vi "SimAcq.vi"(8 "error in (no error)":errorcluster, 11 "Instruments in":refnum<class "Instruments.lvclass">) -> (0 "error out":errorcluster, 3 "Instruments out":refnum<class "Instruments.lvclass">)   [LabVIEW 2012, in "Instruments.lvclass"]
uses:
  Instruments.lvclass
  Controls/TestData.ctl
  Controls/Measurement.ctl
  Controls/CurrentPad.ctl
  Controls/PadArea.ctl
  <userlib>/_OpenG.lib/numeric/numeric.llb/Random Number Within Range - DBL__ogtk.vi
panel:
  in  "Value":T1
  out "TestData":T3 {"50mA Data"."Reverse" format="%#_3g"; "50mA Data"."Current,mA" format="%_6g"; "50mA Data"."Knee Current" format="%#_3g"; "50mA Data"."WL" format="%_6g"; "50mA Data"."Voltage" format="%_6g"; "50mA Data"."Power" format="%_5g"; "20mA Data"."Reverse" format="%#_3g"; "20mA Data"."Current,mA" format="%_6g"; "20mA Data"."Knee Current" format="%#_3g"; "20mA Data"."WL" format="%_6g"; "20mA Data"."Voltage" format="%_6g"; "20mA Data"."Power" format="%_5g"}
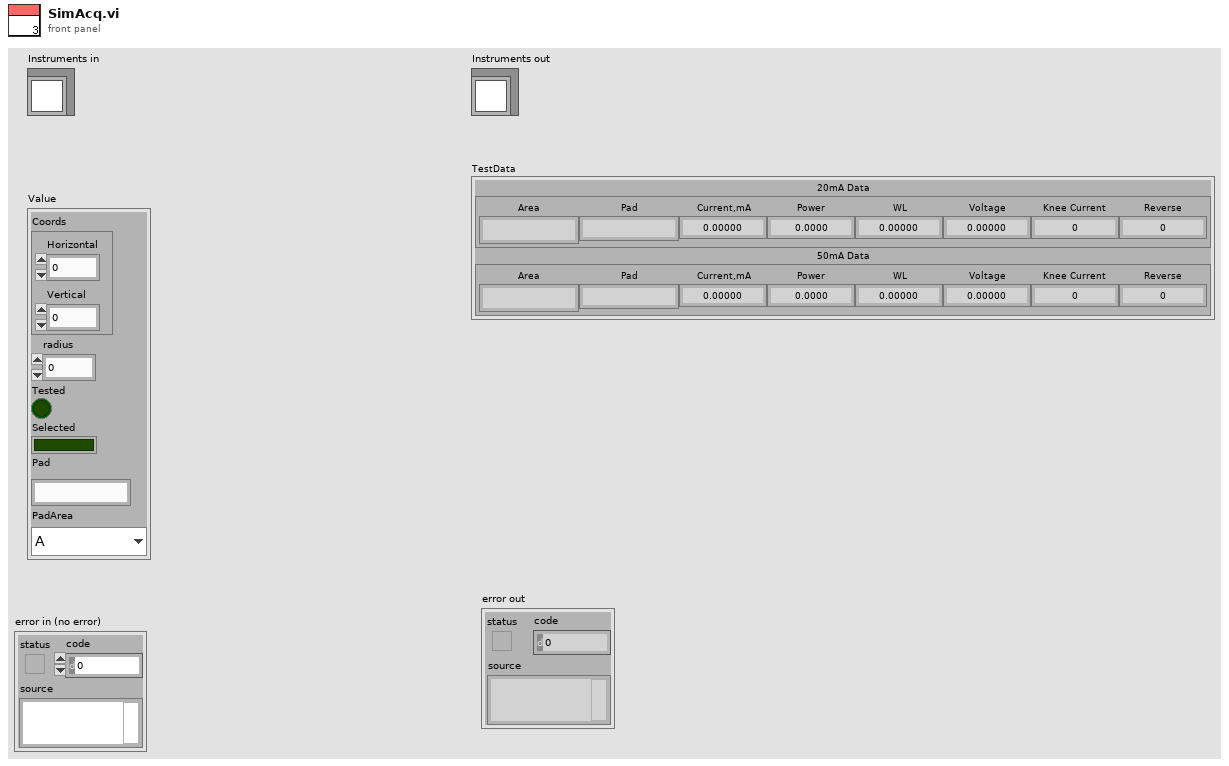
[diagram p1: front panel]
types:
  T1 = typedef "CurrentPad.ctl" = cluster{"Coords":cluster{"Horizontal":sgl, "Vertical":sgl}, "radius":i32, "Tested":bool, "Selected":bool, "Pad":string, "PadArea":T2}
  T2 = typedef "PadArea.ctl" = enum16{"A", "B", "C", "D", "L", "R", "T", "G"}
  T3 = typedef "TestData.ctl" = cluster{"20mA Data":T4, "50mA Data ":T4}
  T4 = typedef "Measurement.ctl" = cluster{"Area":string, "Pad":string, "Current,mA":dbl, "Power":dbl, "WL":dbl, "Voltage":dbl, "Knee Current":dbl, "Reverse":dbl}
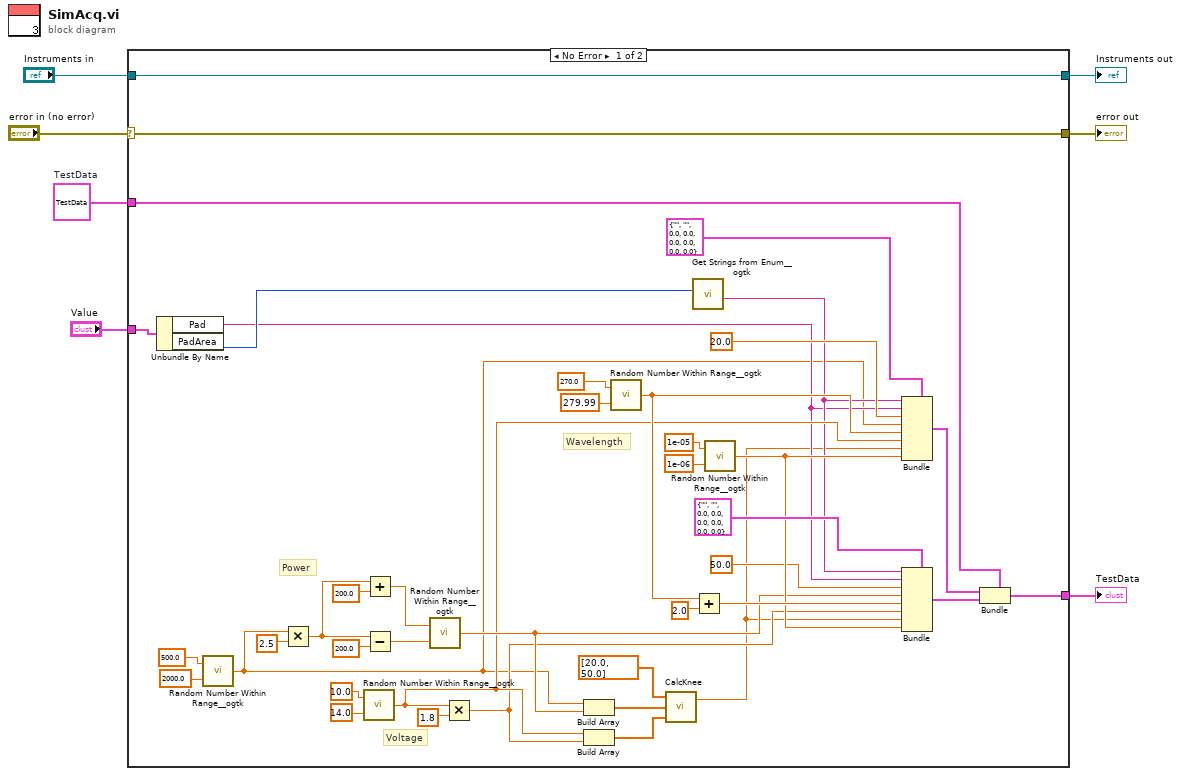
[diagram p0: block diagram]
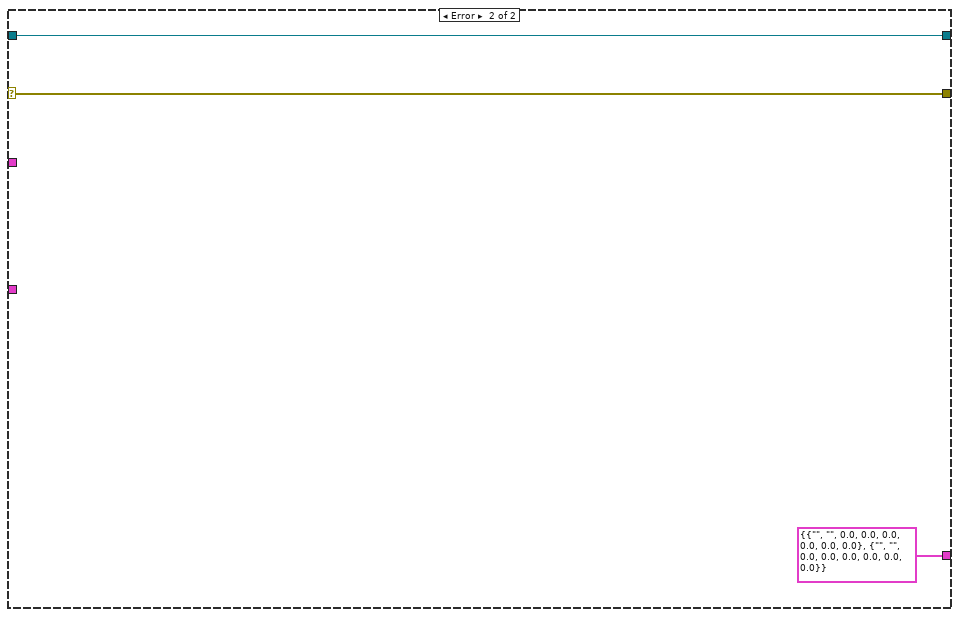
[diagram p2: hidden frame]
diagram:
  w3 = T3 {"20mA Data"={"Area"="", "Pad"="", "Current,mA"=0.0, "Power"=0.0, "WL"=0.0, "Voltage"=0.0, "Knee Current"=0.0, "Reverse"=0.0}, "50mA Data "={"Area"="", "Pad"="", "Current,mA"=0.0, "Power"=0.0, "WL"=0.0, "Voltage"=0.0, "Knee Current"=0.0, "Reverse"=0.0}}  # TestData
  n1 = case shown="No Error" "error in (no error)" {
    selector: "error in (no error)" -> [w48 w51]
    tunnel: [w48 w51] -> w6
    tunnel: [w47 w50] -> w4
    tunnel: "Instruments in" -> [w47 w50]
    tunnel: w3 -> [w46 _]
    tunnel: [w45 T3 {"20mA Data"={"Area"="", "Pad"="", "Current,mA"=0.0, "Power"=0.0, "WL"=0.0, "Voltage"=0.0, "Knee Current"=0.0, "Reverse"=0.0}, "50mA Data "={"Area"="", "Pad"="", "Current,mA"=0.0, "Power"=0.0, "WL"=0.0, "Voltage"=0.0, "Knee Current"=0.0, "Reverse"=0.0}} ("TestData")] -> w2
    tunnel: "Value" -> [w44 _]
    frame No Error {
      # "Wavelength"
      # "Voltage"
      # "Power"
      n2 = Unbundle By Name(w44) -> ("Pad"=w10:string, "PadArea"=w42:T2)
      n3 = call-poly <userlib>:"Random Number Within Range__ogtk.vi"("High"=500.0, "Low"=2000.0) -> ("Random Number"=w8:dbl)  [unwired: 3 in]
      n4 = Multiply(x=w8, y=2.5) -> (x*y=w28:dbl)
      n5 = call-poly <userlib>:"Random Number Within Range__ogtk.vi"("High"=10.0, "Low"=14.0) -> ("Random Number"=w19:dbl)  [unwired: 3 in]
      n6 = Add(x=w28, y=200.0) -> (x+y=w30:dbl)
      n7 = Subtract(x=w28, y=200.0) -> (x-y=w29:dbl)
      n8 = call-poly <userlib>:"Random Number Within Range__ogtk.vi"("High"=w30, "Low"=w29) -> ("Random Number"=w21:dbl)  [unwired: 3 in]
      n9 = Multiply(x=w19, y=1.8) -> (x*y=w18:dbl)
      n10 = Build Array(w8, w21) -> (w20:dbl[])
      n11 = Build Array(w19, w18) -> (w17:dbl[])
      n12 = call-poly <userlib>:"Random Number Within Range__ogtk.vi"("High"=270.0, "Low"=279.99) -> ("Random Number"=w26:dbl)  [unwired: 3 in]
      n13 = call "CalcKnee.vi"("Voltage"=w17, "Power"=w20, "Current"=dbl[] [20.0, 50.0]) -> ("Knee Current"=w9:dbl)  [unwired: 1 out]
      n14 = call <userlib>:"Get Strings from Enum__ogtk.vi"("Enum"=w42) -> ("String Value"=w11:string)  [unwired: 7 in, 3 out]
      n15 = Add(x=w26, y=2.0) -> (x+y=w24:dbl)
      n16 = call-poly <userlib>:"Random Number Within Range__ogtk.vi"("High"=1e-05, "Low"=1e-06) -> ("Random Number"=w22:dbl)  [unwired: 3 in]
      n17 = Bundle(cluster=T4 {"Area"="", "Pad"="", "Current,mA"=0.0, "Power"=0.0, "WL"=0.0, "Voltage"=0.0, "Knee Current"=0.0, "Reverse"=0.0} ("20mA Data"), "Area"=w11, "Pad"=w10, "Current,mA"=20.0, "Power"=w8, "WL"=w26, "Voltage"=w19, "Knee Current"=w9, "Reverse"=w22) -> (w15:T4)
      n18 = Bundle(cluster=T4 {"Area"="", "Pad"="", "Current,mA"=0.0, "Power"=0.0, "WL"=0.0, "Voltage"=0.0, "Knee Current"=0.0, "Reverse"=0.0} ("50mA Data"), "Area"=w11, "Pad"=w10, "Current,mA"=50.0, "Power"=w21, "WL"=w24, "Voltage"=w18, "Knee Current"=w9, "Reverse"=w22) -> (w14:T4)
      n19 = Bundle(cluster=w46, "20mA Data"=w15, "50mA Data"=w14) -> (w45:T3)
    }
    frame Error {
    }
  }
  "error out" <- w6
  "Instruments out" <- w4
  "TestData" <- w2
